vi "SetReverse.vi"(8 "error in (no error)":errorcluster, 10 "Reverse":bool, 11 "Climber in":refnum<class "Climber.lvclass">) -> (0 "error out":errorcluster, 3 "Climber out":refnum<class "Climber.lvclass">)   [LabVIEW 2016, in "Climber.lvclass"]
uses:
  Climber.lvclass
  Climber.lvclass/Climber.ctl
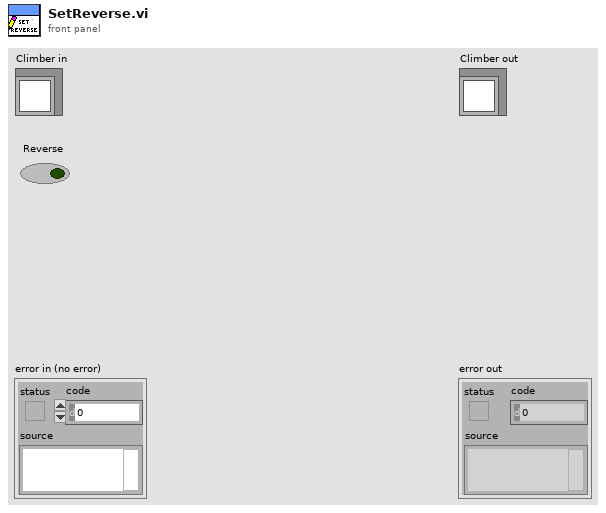
[diagram p1: front panel]
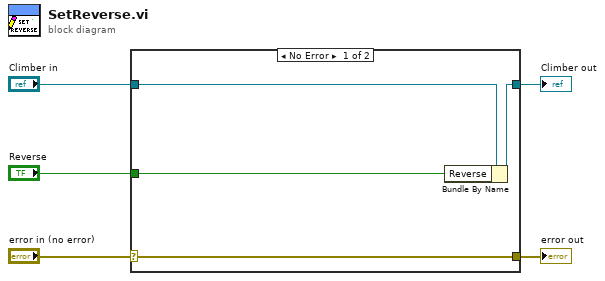
[diagram p0: block diagram]
diagram:
  n1 = case shown="No Error" "error in (no error)" {
    selector: "error in (no error)" -> [w9 w10]
    tunnel: [w9 w10] -> w4
    tunnel: [w7 w11] -> w2
    tunnel: "Climber in" -> [w8 w11]
    tunnel: "Reverse" -> [w6 _]
    frame No Error {
      n2 = Bundle By Name(cluster=w8, "Reverse"=w6) -> (w7:refnum<class "Climber.lvclass">)
    }
    frame Error {
    }
  }
  "error out" <- w4
  "Climber out" <- w2
